vi "Loop Timing example.vi"() -> ()   [LabVIEW 2020]
panel:
  out "Loop 3 exit":bool
  out "Arbitary start ime":u32
  out "relative time":u32
  out "Loop 2 exit":bool
  out "Loop  1 exit":bool
  in  "Exit":bool
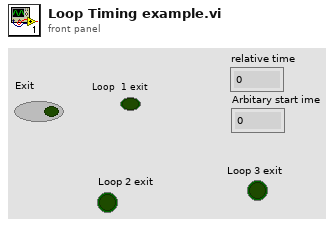
[diagram p1: front panel]
types:
  T1 = typedef "Rendezvous RefNum" = refnum<k1>
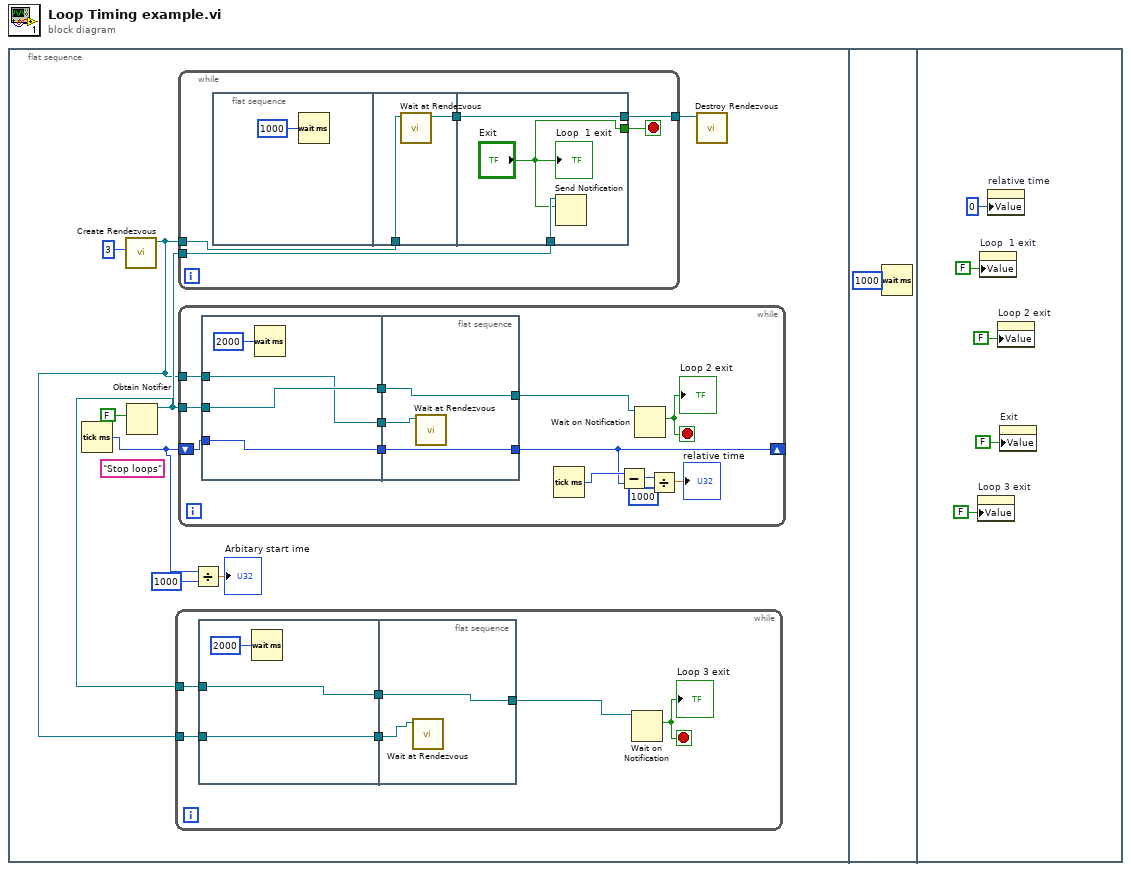
[diagram p0: block diagram]
diagram:
  n1 = flat-sequence {
    frame #0 {
      (unwired) "Stop loops" ("name (unnamed)")
      n2 = Tick Count (ms)() -> (millisecond timer value=w4:u32)
      n3 = call <vilib>:"Create Rendezvous.vi"("size (2)"=3) -> ("rendezvous"=w1:T1)  [unwired: 4 in, 2 out]
      n4 = Obtain Notifier(notification data type=FALSE) -> (notifier out=w2:refnum<notifier>)  [unwired: 3 in, 2 out]
      n5 = while {
        tunnel: w2 -> [w11]
        tunnel: w1 -> [w9]
        stop <- w14 stop-if-true
        n6 = flat-sequence {
          tunnel: [w16] -> w12
          tunnel: w11 -> [w16]
          tunnel: [w15] -> w10
          tunnel: w9 -> [w15]
          tunnel: [w19] -> w13
          tunnel: w12 -> [w19]
          tunnel: w10 -> [w18]
          frame #0 {
            n7 = Wait (ms)(milliseconds to wait=u32 2000) -> ()  [unwired: 1 out]
          }
          frame #1 {
            n8 = call <vilib>:"Wait at Rendezvous.vi"("rendezvous"=w18) -> ()  [unwired: 4 in, 3 out]
          }
        }
        n9 = Wait on Notification(notifier=w13) -> (notification=w14:bool)  [unwired: 3 in, 3 out]
        "Loop 3 exit" <- w14
      }
      n10 = while {
        tunnel: w2 -> [w41]
        tunnel: w1 -> [w44]
        tunnel: [w43] -> w6
        stop <- w40 stop-if-true
        n11 = flat-sequence {
          tunnel: w44 -> [w47]
          tunnel: [w46] -> w42
          tunnel: [w50] -> w43
          tunnel: w42 -> [w50]
          tunnel: w41 -> [w49]
          tunnel: ["Exit"] -> w40
          frame #0 {
            n12 = Wait (ms)(milliseconds to wait=u32 1000) -> ()  [unwired: 1 out]
          }
          frame #1 {
            n13 = call <vilib>:"Wait at Rendezvous.vi"("rendezvous"=w47) -> ("rendezvous out"=w46:T1)  [unwired: 4 in, 2 out]
          }
          frame #2 {
            n14 = Send Notification(notification="Exit", notifier=w49) -> ()  [unwired: 1 in, 2 out]
            "Loop  1 exit" <- "Exit"
          }
        }
      }
      n15 = while {
        tunnel: w2 -> [w29]
        tunnel: w1 -> [w27]
        shift-right: [w20] -> _
        shift-left: w4 -> [w25]
        stop <- w32 stop-if-true
        n16 = flat-sequence {
          tunnel: [w35] -> w30
          tunnel: w29 -> [w35]
          tunnel: [w34] -> w28
          tunnel: w27 -> [w34]
          tunnel: [w33] -> w26
          tunnel: w25 -> [w33]
          tunnel: [w39] -> w31
          tunnel: w30 -> [w39]
          tunnel: w28 -> [w38]
          tunnel: [w37] -> w20
          tunnel: w26 -> [w37]
          frame #0 {
            n17 = Wait (ms)(milliseconds to wait=u32 2000) -> ()  [unwired: 1 out]
          }
          frame #1 {
            n18 = call <vilib>:"Wait at Rendezvous.vi"("rendezvous"=w38) -> ()  [unwired: 4 in, 3 out]
          }
        }
        n19 = Tick Count (ms)() -> (millisecond timer value=w21:u32)
        n20 = Subtract(x=w21, y=w20) -> (x-y=w23:u32)
        n21 = Wait on Notification(notifier=w31) -> (notification=w32:bool)  [unwired: 3 in, 3 out]
        "Loop 2 exit" <- w32
        n22 = Divide(x=w23, y=u32 1000) -> (x/y=→"relative time":dbl)
      }
      n23 = Divide(x=w4, y=u32 1000) -> (x/y=→"Arbitary start ime":dbl)
      n24 = call <vilib>:"Destroy Rendezvous.vi"("rendezvous"=w6) -> ()  [unwired: 5 in, 2 out]
    }
    frame #1 {
      n25 = Wait (ms)(milliseconds to wait=u32 1000) -> ()  [unwired: 1 out]
    }
    frame #2 {
      n26 = property on="Loop 3 exit" class="Bool (strict)"("Value"=FALSE ("Loop 3 exit")) -> ()  [unwired: 2 in, 2 out]
      n27 = property on="Loop  1 exit" class="Bool (strict)"("Value"=FALSE ("Loop  1 exit")) -> ()  [unwired: 2 in, 2 out]
      n28 = property on="relative time" class="DigNum (strict)"("Value"=u32 0 ("relative time")) -> ()  [unwired: 2 in, 2 out]
      n29 = property on="Loop 2 exit" class="Bool (strict)"("Value"=FALSE ("Boolean 3")) -> ()  [unwired: 2 in, 2 out]
      n30 = property on="Exit" class="Bool (strict)"("Value"=FALSE ("Exit")) -> ()  [unwired: 2 in, 2 out]
    }
  }
